vi "基于Labview和CAN总线的电机监控系统.vi"() -> ()   [LabVIEW 2012]
uses:
  <vilib>/nican/nicantsk.llb/CAN Interface.ctl
  <vilib>/nican/nicantsk.llb/CAN Write Multi Chan Single Samp 1D Dbl.vi
  <vilib>/Utility/file.llb/Write To Spreadsheet File (DBL).vi
  <vilib>/nican/nicantsk.llb/CAN Read Multi Chan Multi Samp 2D Dbl.vi
  <vilib>/measure/NI_MABase.lvlib
panel:
  in  "仿真":bool=TRUE
  in  "报文ID":string
  out "时间":string
  in  "关闭电机":bool
  in  "停止运动":bool
  in  "开始运动":bool
  in  "转动方向":bool
  in  "历史数据":bool
  in  "目标转速（r/min）":dbl=600.0
  in  "参数设置":bool
  out "转速波形":dbl[](graph)
  out "电流波形":dbl[](graph)
  out "电压波形":dbl[](graph)
  in  "文件名":string="电机参数"
  in  "数据存储路径":path=path "E:/数据保存"
  in  "退出":bool
  out "当前转速":dbl
  out "当前电流":dbl
  out "当前电压":dbl
  in  "最高转速(r/min)":dbl=5000.0
  in  "最大电流(A)":dbl=4.0
  in  "最大电压(V)":dbl=320.0
  in  "微分常数":dbl=0.01
  in  "积分常数":dbl=0.2
  in  "比例常数":dbl=3.0
  out "超速":bool
  out "过流":bool
  out "过压":bool
  in  "关闭CAN连接":bool
  in  "启动CAN连接":bool
  in  "interface":T1=64 items=["CAN0"=0, "CAN1"=1, "CAN2"=2, "CAN3"=3, "CAN4"=4, "CAN5"=5, "CAN6"=6, "CAN7"=7, "CAN8"=8, "CAN9"=9, "CAN10"=10, "CAN11"=11, "CAN12"=12, "CAN13"=13, "CAN14"=14, "CAN15"=15, "CAN16"=16, "CAN17"=17, "CAN18"=18, "CAN19"=19, "CAN20"=20, "CAN21"=21, "CAN22"=22, "CAN23"=23, "CAN24"=24, "CAN25"=25, "CAN26"=26, "CAN27"=27, "CAN28"=28, "CAN29"=29, "CAN30"=30, "CAN31"=31, "CAN32"=32, "CAN33"=33, "CAN34"=34, "CAN35"=35, "CAN36"=36, "CAN37"=37, "CAN38"=38, "CAN39"=39, "CAN40"=40, "CAN41"=41, "CAN42"=42, "CAN43"=43, "CAN44"=44, "CAN45"=45, "CAN46"=46, "CAN47"=47, "CAN48"=48, "CAN49"=49, "CAN50"=50, "CAN51"=51, "CAN52"=52, "CAN53"=53, "CAN54"=54, "CAN55"=55, "CAN56"=56, "CAN57"=57, "CAN58"=58, "CAN59"=59, "CAN60"=60, "CAN61"=61, "CAN62"=62, "CAN63"=63, "MAX default"=64, "CAN256 (Virtual)"=256, "CAN257 (Virtual)"=257]
  in  "sample rate":dbl format="%.2f"
  # "基于Labview和CAN总线的电机监控系统"
  # "CAN硬件配置"
  # "报警上限配置"
  # "PID参数设置"
  # "反向"
  # "正向"
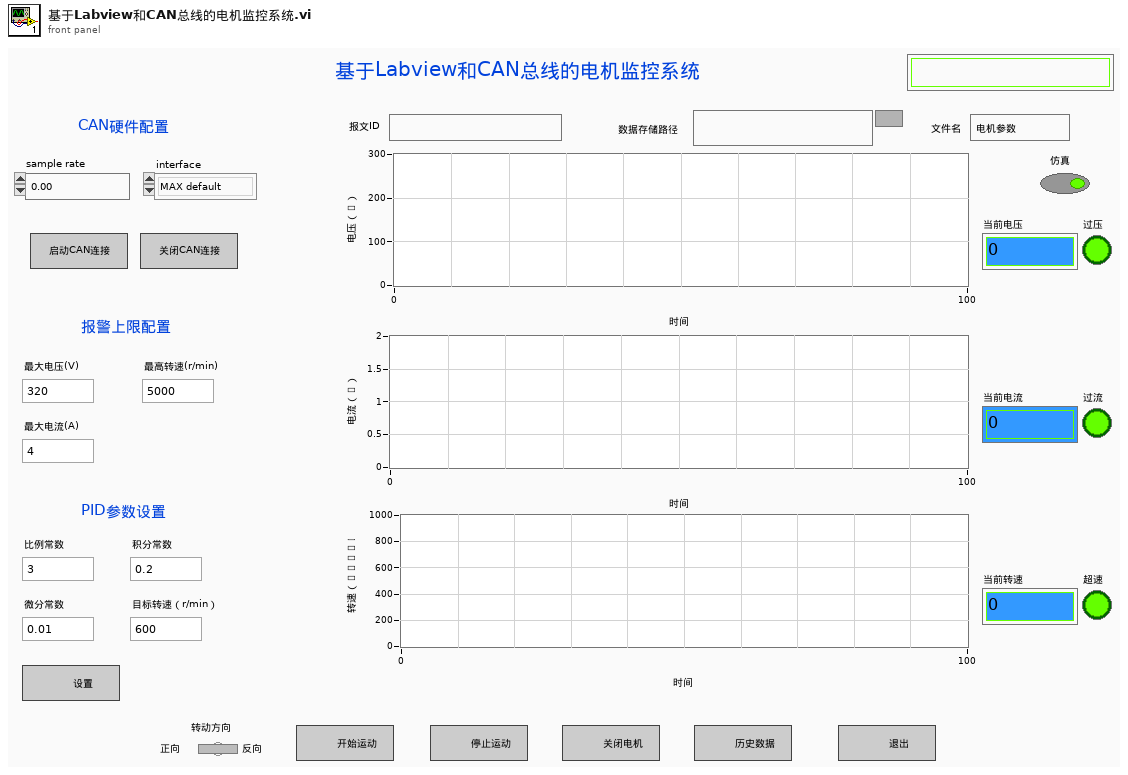
[diagram p1: front panel]
types:
  T1 = typedef "CAN Interface.ctl" = u16
  T2 = typedef "CAN Task Reference.ctl" = u32
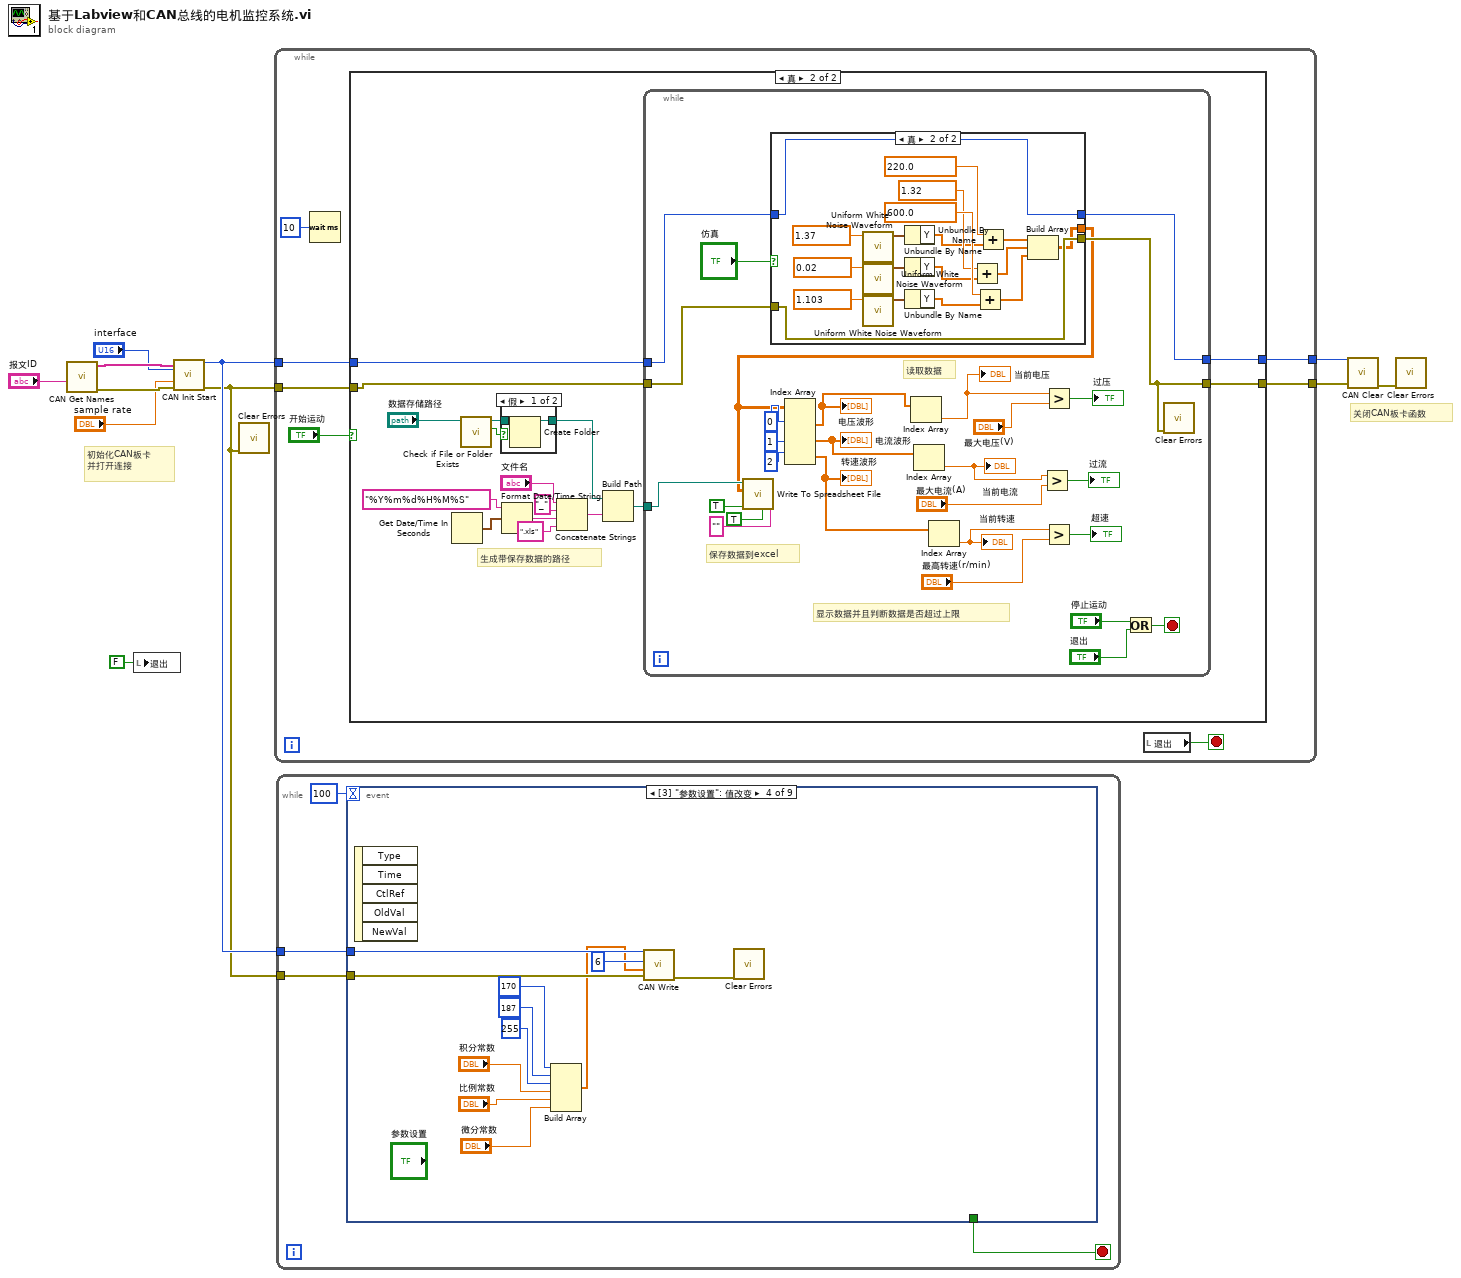
[diagram p0: block diagram]
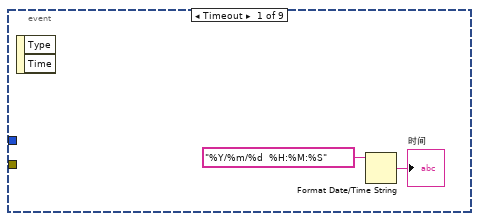
[diagram p2: hidden frame]
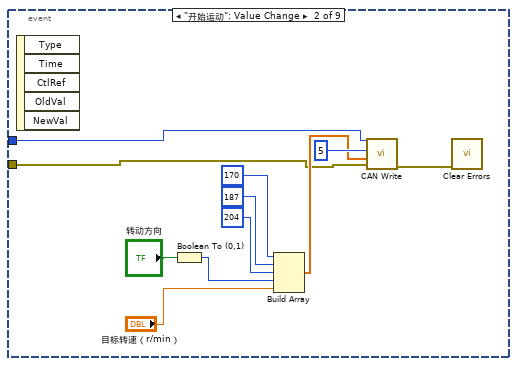
[diagram p3: hidden frame]
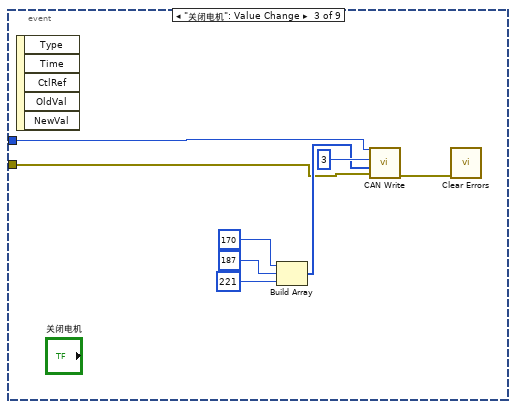
[diagram p4: hidden frame]
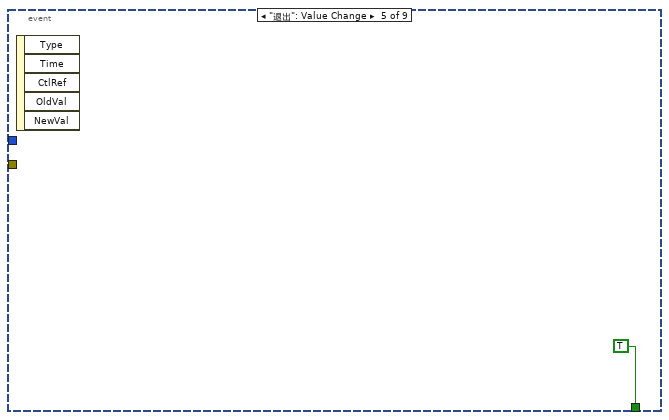
[diagram p5: hidden frame]
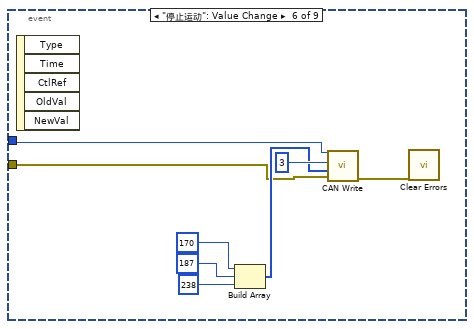
[diagram p6: hidden frame]
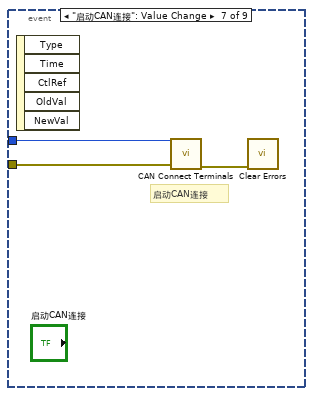
[diagram p7: hidden frame]
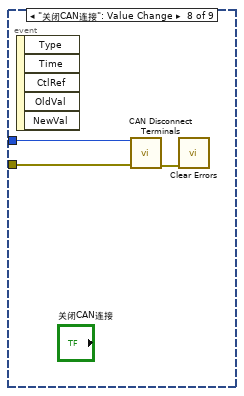
[diagram p8: hidden frame]
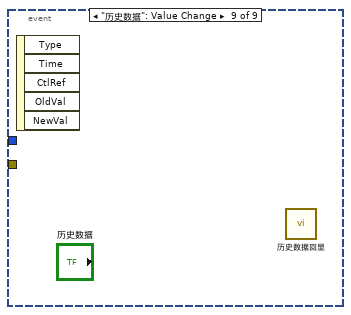
[diagram p9: hidden frame]
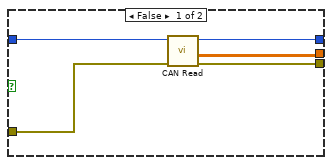
[diagram p12: hidden frame]
diagram:
  # "关闭CAN板卡函数"
  # "初始化CAN板卡\n并打开连接"
  n1 = call <vilib>:"CAN Get Names.vi"("message name"="报文ID") -> ("error out"=w10:errorcluster, "channel list"=w11:string[])  [unwired: 9 in]
  n2 = local write "退出"(FALSE ("退出")) -> ()
  n3 = call <vilib>:"CAN Init Start.vi"("channel list"=w11, "interface"="interface", "sample rate"="sample rate", "error in (no error)"=w10) -> ("task reference out"=w5:T2, "error out"=w2:errorcluster)  [unwired: 10 in]
  n4 = call <vilib>:"Clear Errors.vi"("error in (no error)"=w2) -> ()  [unwired: 6 in, 1 out]
  n5 = while {
    tunnel: w5 -> [w18]
    tunnel: w2 -> [w17]
    tunnel: [w16] -> w7
    tunnel: [w15] -> w6
    stop <- w13 stop-if-true
    n6 = Wait (ms)(milliseconds to wait=u32 10 ("等待时间（毫秒）")) -> ()  [unwired: 1 out]
    n7 = case shown="真" "开始运动" {
      tunnel: w18 -> [w20 w36]
      tunnel: w17 -> [w19 w35]
      tunnel: [w20 w34] -> w16
      tunnel: [w19 w33] -> w15
      frame False {
      }
      frame True {
        # "生成带保存数据的路径"
        n8 = Get Date/Time In Seconds() -> (seconds since 1Jan1904=w32:timestamp)
        n9 = call <vilib>:"Check if File or Folder Exists.vi"("path"="数据存储路径") -> ("file or folder exists?"=w25:bool, "dup path"=w24:path)  [unwired: 8 in, 1 out]
        n10 = case shown="假" w25 {
          tunnel: w24 -> [w38 w39]
          tunnel: [w37 w39] -> w23
          frame False {
            n11 = Create Folder(path (use dialog)=w38) -> (created path=w37:path)  [unwired: 2 in, 2 out]
          }
          frame True {
          }
        }
        n12 = Format Date/Time String(time format string (%c)="%Y%m%d%H%M%S" ("时间格式字符串(%c)"), seconds (now)=w32) -> (date/time string=w27:string)  [unwired: 1 in]
        n13 = Concatenate Strings("文件名", "_", w27, ".xls" ("字符串")) -> (w30:string)
        n14 = Build Path(base path=w23, name or relative path=w30) -> (appended path=w21:path)
        n15 = while {
          tunnel: w36 -> [w44]
          tunnel: w35 -> [w43]
          tunnel: [w42] -> w34
          tunnel: [w41] -> w33
          tunnel: w21 -> [w64]
          stop <- w55 stop-if-true
          # "显示数据并且判断数据是否超过上限"
          # "读取数据"
          # "保存数据到excel"
          n16 = case shown="真" "仿真" {
            tunnel: w44 -> [w72 w75]
            tunnel: w43 -> [w71 w74]
            tunnel: [w70 w75] -> w42
            tunnel: [w69 w74] -> w41
            tunnel: [w68 w73] -> w40
            frame False {
              n17 = call-poly <vilib>:"CAN Read.vi"("error in (no error)"=w71, "task reference in"=w72) -> ("error out"=w69:errorcluster, "multi-chan multi-samp 2D dbl"=w68:dbl[][], "task reference out"=w70:T2)  [unwired: 6 in, 1 out]
            }
            frame True {
              n18 = call <vilib>:"Uniform White Noise Waveform.vi"("amplitude"=1.37) -> ("signal out"=w82:waveform(dbl))  [unwired: 9 in, 1 out]
              n19 = call <vilib>:"Uniform White Noise Waveform.vi"("amplitude"=0.02) -> ("signal out"=w83:waveform(dbl))  [unwired: 9 in, 1 out]
              n20 = call <vilib>:"Uniform White Noise Waveform.vi"("amplitude"=1.103) -> ("signal out"=w84:waveform(dbl))  [unwired: 9 in, 1 out]
              n21 = Unbundle By Name(w82) -> ("Y"=w87:dbl[])
              n22 = Unbundle By Name(w83) -> ("Y"=w86:dbl[])
              n23 = Unbundle By Name(w84) -> ("Y"=w85:dbl[])
              n24 = Add(x=1.32 ("amplitude"), y=w86) -> (x+y=w77:dbl[])
              n25 = Add(x=600.0 ("amplitude"), y=w85) -> (x+y=w76:dbl[])
              n26 = Add(x=220.0 ("amplitude"), y=w87) -> (x+y=w78:dbl[])
              n27 = Build Array(w78, w77, w76) -> (w73:dbl[][])
            }
          }
          n28 = call-poly <vilib>:"Write To Spreadsheet File.vi"("delimiter (\\t)"="" ("delimiter (\\t)"), "transpose? (no:F)"=TRUE, "append to file? (new file:F)"=TRUE, "2D data"=w40, "file path (dialog if empty)"=w64) -> ()  [unwired: 3 in, 1 out]
          n29 = Index Array(array=w40, index (row) #1=0 ("索引 (行)"), index (row) #2=1 ("索引 (行)"), index (row) #3=2 ("索引 (行)")) -> (element #1=w60:dbl[], element #2=w59:dbl[], element #3=w58:dbl[])  [unwired: 3 in]
          "电流波形" <- w59
          "电压波形" <- w60
          "转速波形" <- w58
          n30 = Index Array(array=w60) -> (element=w54:dbl)  [unwired: 1 in]
          "当前电压" <- w54
          n31 = Index Array(array=w59) -> (element=w52:dbl)  [unwired: 1 in]
          "当前电流" <- w52
          n32 = Index Array(array=w58) -> (element=w51:dbl)  [unwired: 1 in]
          "当前转速" <- w51
          n33 = Greater?(x=w52, y="最大电流(A)") -> (0:→"过流":bool)
          n34 = Greater?(x=w54, y="最大电压(V)") -> (0:→"过压":bool)
          n35 = Greater?(x=w51, y="最高转速(r/min)") -> (0:→"超速":bool)
          n36 = Or(x="停止运动", y="退出") -> (x .or. y?=w55:bool)
          n37 = call <vilib>:"Clear Errors.vi"("error in (no error)"=w41) -> ()  [unwired: 6 in, 1 out]
        }
      }
    }
    n38 = local read "退出"() -> (w13:bool)
  }
  n39 = while {
    tunnel: w5 -> [w93]
    tunnel: w2 -> [w92]
    stop <- w91 stop-if-true
    n40 = event shown="[3] \"参数设置\": 值改变" {
      selector: _ -> [_ _ _ _ _ _ _ _ _]
      dyn-events: _ -> [_ _ _ _ _ _ _ _ _]
      timeout: 100 -> [_ _ _ _ _ _ _ _ _]
      tunnel: w93 -> [_ w102 w110 w126 _ w130 w138 w141 _]
      tunnel: w92 -> [_ w101 w109 w125 _ w129 w137 w140 _]
      tunnel: [_ _ _ _ TRUE ("参数设置 2") _ _ _ _] -> w91
      event Timeout {
        n41 = event-data() -> ()  [unwired: 1 in, 2 out]
        n42 = Format Date/Time String(time format string (%c)="%Y/%m/%d  %H:%M:%S" ("时间格式字符串(%c)")) -> (date/time string=→"时间":string)  [unwired: 2 in]
      }
      event "开始运动": Value Change {
        n43 = event-data() -> ()  [unwired: 1 in, 5 out]
        n44 = Boolean To (0,1)(Boolean="转动方向") -> (0, 1=w99:i16)
        n45 = Build Array(u16 170 ("元素"), u16 187 ("元素"), u16 204 ("元素"), w99, "目标转速（r/min）") -> (w106:dbl[])
        n46 = call-poly <vilib>:"CAN Write.vi"("error in (no error)"=w101, "multi-chan single-samp 1D dbl"=w106, "number of samples to write"=u32 5, "task reference in"=w102) -> ("error out"=w97:errorcluster)  [unwired: 6 in, 1 out]
        n47 = call <vilib>:"Clear Errors.vi"("error in (no error)"=w97) -> ()  [unwired: 6 in, 1 out]
      }
      event "关闭电机": Value Change {
        n48 = event-data() -> ()  [unwired: 1 in, 5 out]
        n49 = Build Array(u16 170 ("元素"), u16 187 ("元素"), u16 221 ("元素")) -> (w114:u16[])
        n50 = call-poly <vilib>:"CAN Write.vi"("error in (no error)"=w109, "multi-chan single-samp 1D dbl"=w114, "number of samples to write"=u32 3, "task reference in"=w110) -> ("error out"=w108:errorcluster)  [unwired: 6 in, 1 out]
        n51 = call <vilib>:"Clear Errors.vi"("error in (no error)"=w108) -> ()  [unwired: 6 in, 1 out]
      }
      event "参数设置": Value Change {
        n52 = event-data() -> ()  [unwired: 1 in, 5 out]
        n53 = Build Array(u16 170 ("元素"), u16 187 ("元素"), u16 255 ("元素"), "积分常数", "比例常数", "微分常数") -> (w120:dbl[])
        n54 = call-poly <vilib>:"CAN Write.vi"("error in (no error)"=w125, "multi-chan single-samp 1D dbl"=w120, "number of samples to write"=u32 6, "task reference in"=w126) -> ("error out"=w116:errorcluster)  [unwired: 6 in, 1 out]
        n55 = call <vilib>:"Clear Errors.vi"("error in (no error)"=w116) -> ()  [unwired: 6 in, 1 out]
      }
      event "退出": Value Change {
        n56 = event-data() -> ()  [unwired: 1 in, 5 out]
      }
      event "停止运动": Value Change {
        n57 = event-data() -> ()  [unwired: 1 in, 5 out]
        n58 = Build Array(u16 170 ("元素"), u16 187 ("元素"), u16 238 ("元素")) -> (w134:u16[])
        n59 = call-poly <vilib>:"CAN Write.vi"("error in (no error)"=w129, "multi-chan single-samp 1D dbl"=w134, "number of samples to write"=u32 3, "task reference in"=w130) -> ("error out"=w128:errorcluster)  [unwired: 6 in, 1 out]
        n60 = call <vilib>:"Clear Errors.vi"("error in (no error)"=w128) -> ()  [unwired: 6 in, 1 out]
      }
      event "启动CAN连接": Value Change {
        # "启动CAN连接"
        n61 = event-data() -> ()  [unwired: 1 in, 5 out]
        n62 = call <vilib>:"CAN Connect Terminals.vi"("error in (no error)"=w137, "task reference in"=w138) -> ("error out"=w136:errorcluster)  [unwired: 8 in, 1 out]
        n63 = call <vilib>:"Clear Errors.vi"("error in (no error)"=w136) -> ()  [unwired: 6 in, 1 out]
      }
      event "关闭CAN连接": Value Change {
        n64 = event-data() -> ()  [unwired: 1 in, 5 out]
        n65 = call <vilib>:"CAN Disconnect Terminals.vi"("error in (no error)"=w140, "task reference in"=w141) -> ("error out"=w139:errorcluster)  [unwired: 8 in, 1 out]
        n66 = call <vilib>:"Clear Errors.vi"("error in (no error)"=w139) -> ()  [unwired: 6 in, 1 out]
      }
      event "历史数据": Value Change {
        n67 = event-data() -> ()  [unwired: 1 in, 5 out]
        n68 = call "历史数据回显.vi"() -> ()  [unwired: 12 in]
      }
    }
  }
  n69 = call <vilib>:"CAN Clear.vi"("error in (no error)"=w6, "task reference in"=w7) -> ("error out"=w3:errorcluster)  [unwired: 9 in]
  n70 = call <vilib>:"Clear Errors.vi"("error in (no error)"=w3) -> ()  [unwired: 6 in, 1 out]
